vi "init.vi"(8 "error in (no error)":errorcluster, 11 "coffe actor in":refnum<class "coffe actor.lvclass">) -> (0 "error out":errorcluster, 3 "coffe actor out":refnum<class "coffe actor.lvclass">)   [LabVIEW 2020, in "coffe actor.lvlib" / "coffe actor.lvclass"]
uses:
  coffe actor.lvclass
  coffe actor.lvclass/coffe actor.ctl
  <vilib>/Utility/config.llb/Read Key (Double).vi
  <vilib>/Utility/config.llb/Read Key (String).vi
  <vilib>/Utility/config.llb/NI_LVConfig.lvlib
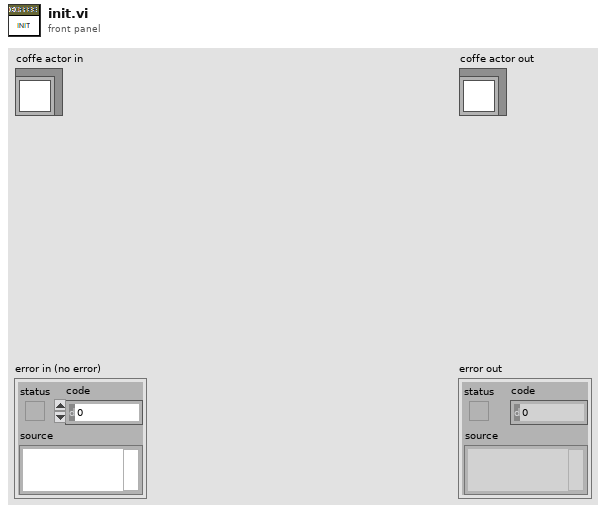
[diagram p1: front panel]
types:
  T1 = typedef "NI_LVConfig.lvlib/Config Data RefNum.ctl" = refnum<k1>
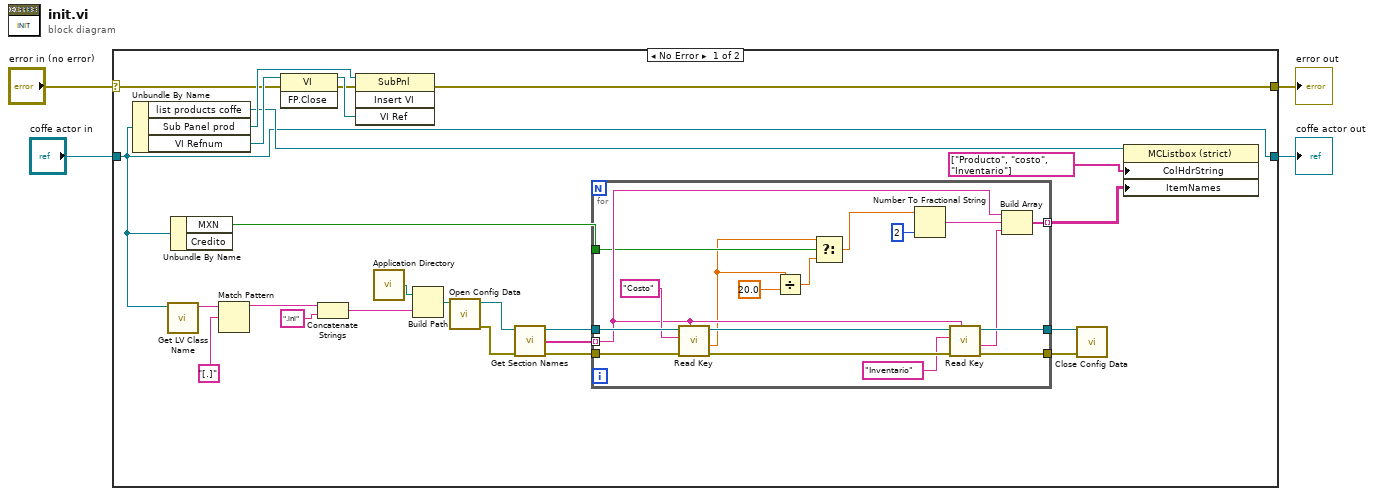
[diagram p0: block diagram]
diagram:
  n1 = case shown="No Error" "error in (no error)" {
    selector: "error in (no error)" -> [w25 w49]
    tunnel: [w24 w49] -> w3
    tunnel: [w14 w48] -> w1
    tunnel: "coffe actor in" -> [w14 w48]
    frame No Error {
      n2 = Unbundle By Name(w14) -> ("list products coffe"=w23:refnum<vi>, "Sub Panel prod"=w29:refnum<vi>, "VI Refnum"=w28:refnum<vi>)
      n3 = call <vilib>:"Get LV Class Name.vi"("object"=w14) -> ("class name"=w17:string)  [unwired: 9 in, 1 out]
      n4 = Unbundle By Name(w14) -> ("MXN"=w13:bool)  [unwired: 1 out]
      n5 = Match Pattern(string=w17, regular expression="[.]") -> (before substring=w15:string)  [unwired: 1 in, 3 out]
      n6 = invoke class="VI" method="FP.Close"(reference=w28, error in=w25) -> (reference out=w27:refnum<vi>, error out=w26:errorcluster)  [unwired: 1 in, 1 out]
      n7 = Concatenate Strings(w15, ".ini" ("string")) -> (w19:string)
      n8 = invoke class="SubPnl" method="Insert VI"(reference=w29, error in=w26, "VI Ref"=w27) -> (error out=w24:errorcluster)  [unwired: 1 in, 3 out]
      n9 = call <vilib>:"Application Directory.vi"() -> ("Application Directory"=w21:path)
      n10 = Build Path(base path=w21, name or relative path=w19) -> (appended path=w18:path)
      n11 = call <vilib>:"Open Config Data.vi"("configuration file path"=w18) -> ("error out"=w12:errorcluster, "refnum"=w11:T1)  [unwired: 8 in, 1 out]
      n12 = call <vilib>:"Get Section Names.vi"("error in (no error)"=w12, "refnum"=w11) -> ("error out"=w9:errorcluster, "section names"=w8:string[], "refnum out"=w10:T1)  [unwired: 7 in]
      n13 = for {
        tunnel: w10 -> [w47]
        tunnel: w9 -> [w46]
        tunnel: [w43] -> w7
        tunnel: [w42] -> w6
        tunnel: w13 -> [w34]
        tunnel: w8 -> [w39] mode=indexing
        tunnel: [w37] -> w5 mode=indexing
        n14 = call-poly <vilib>:"Read Key.vi"("section"=w39, "error in (no error)"=w46, "key"="Costo", "refnum"=w47) -> ("error out"=w45:errorcluster, "value"=w32:dbl, "refnum out"=w44:T1)  [unwired: 4 in, 1 out]
        n15 = Divide(x=w32, y=20.0) -> (x/y=w30:dbl)
        n16 = Select(t=w32, s=w34, f=w30) -> (s? t:f=w33:dbl)
        n17 = Number To Fractional String(number=w33, precision (6)=i16 2) -> (F-format string=w36:string)  [unwired: 2 in]
        n18 = call-poly <vilib>:"Read Key.vi"("section"=w39, "error in (no error)"=w45, "key"="Inventario", "refnum"=w44) -> ("error out"=w43:errorcluster, "value"=w38:string, "refnum out"=w42:T1)  [unwired: 4 in, 1 out]
        n19 = Build Array(w39, w36, w38) -> (w37:string[])
      }
      n20 = call <vilib>:"Close Config Data.vi"("error in (no error)"=w7, "refnum"=w6) -> ()  [unwired: 8 in, 2 out]
      n21 = property class="MCListbox (strict)"(reference=w23, "ColHdrString"=string[] ["Producto", "costo", "Inventario"] ("Column Header Strings[]"), "ItemNames"=w5) -> ()  [unwired: 1 in, 2 out]
    }
    frame Error {
    }
  }
  "error out" <- w3
  "coffe actor out" <- w1
